vi "Timed One-Shot (SubVI).vi"(0 "Trigger Input Pulse":bool, 2 "Reset Signal Output":bool, 5 "ON Time (ms)":dbl=600.0) -> (14 "Signal Output":bool)   [LabVIEW 2009]
panel:
  # "Timed One-Shot (SubVI)\nCreated by Blake Otting\n4/15/2010"
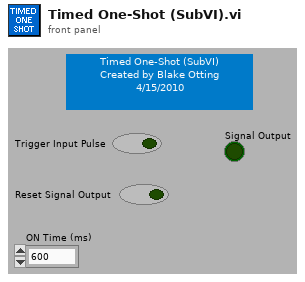
[diagram p1: front panel]
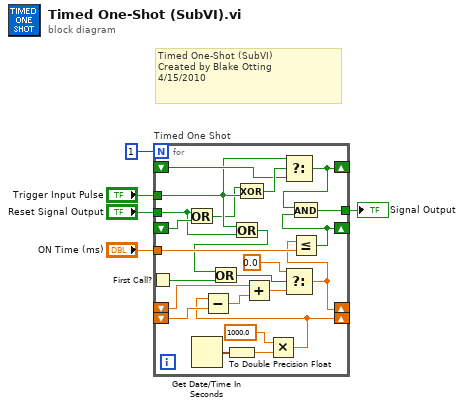
[diagram p0: block diagram]
diagram:
  # "Timed One-Shot (SubVI)\nCreated by Blake Otting\n4/15/2010"
  n1 = for "Timed One Shot" {
    N: 1 -> [_]
    shift-right: [w13] -> _
    shift-left: _ -> [w28]
    shift-right: [w16] -> _
    shift-left: _ -> [w26]
    tunnel: "Trigger Input Pulse" -> [w9]
    shift-right: [w12] -> _
    shift-left: _ -> [w22]
    tunnel: "Reset Signal Output" -> [w6]
    tunnel: "ON Time (ms)" -> [w15]
    shift-right: [w11] -> _
    shift-left: _ -> [w17]
    tunnel: [w10] -> w5
    n2 = First Call?() -> (First Call?: T/F=w21:bool)
    n3 = Or(x=w6, y=w17) -> (x .or. y?=w8:bool)
    n4 = Get Date/Time In Seconds() -> (seconds since 1Jan1904=w27:timestamp)
    n5 = To Double Precision Float(number=w27) -> (double precision float=w18:dbl)
    n6 = Or(x=w9, y=w6) -> (x .or. y?=w7:bool)
    n7 = Or(x=w7, y=w21) -> (x .or. y?=w20:bool)
    n8 = Exclusive Or(1:w9, 2:w8) -> (0:w23:bool)
    n9 = Multiply(x=1000.0, y=w18) -> (x*y=w16:dbl)
    n10 = Subtract(x=w16, y=w26) -> (x-y=w25:dbl)
    n11 = Add(x=w28, y=w25) -> (x+y=w14:dbl)
    n12 = Select(t=w9, s=w23, f=w22) -> (s? t:f=w12:bool)
    n13 = Select(t=0.0, s=w20, f=w14) -> (s? t:f=w13:dbl)
    n14 = Less Or Equal?(x=w13, y=w15) -> (x <= y?=w11:bool)
    n15 = And(x=w12, y=w11) -> (x .and. y?=w10:bool)
  }
  "Signal Output" <- w5
